vi "HDF5_LogTime.vi"(8 "error in (no error)":errorcluster, 9 "Timestamp":dbl, 10 "TimeStamp_dset":T1 format="%.0x") -> (0 "error out":errorcluster, 2 "date/time string":string, 3 "current time":timestamp)   [LabVIEW 2018]
uses:
  <vilib>/addons/h5labview2/base/hid_t.ctl
  lib_path_mod_20200519.vi
  <vilib>/addons/h5labview2/base/H5Equery.vi
  <vilib>/addons/h5labview2/dataset/H5Dwrite.llb/H5Dwrite.xnode
  <vilib>/addons/h5labview2/dataset/H5D.lvlib
  <vilib>/addons/h5labview2/space/H5S.lvlib
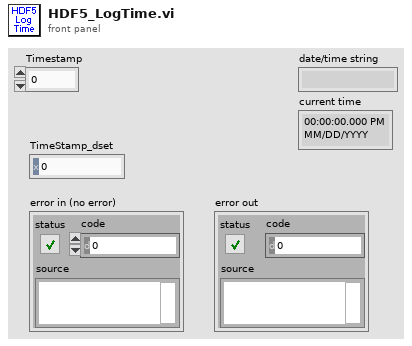
[diagram p1: front panel]
types:
  T1 = typedef "hid_t.ctl" = i32
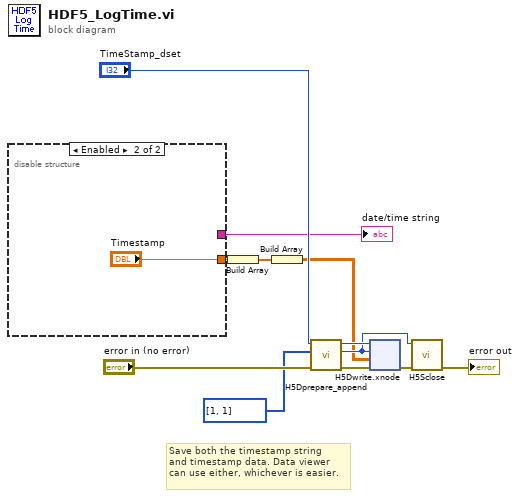
[diagram p0: block diagram]
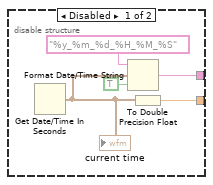
[diagram p2: hidden frame]
diagram:
  # "Save both the timestamp string\nand timestamp data. Data viewer\ncan use either, whichever is easier."
  n1 = disable-structure shown="Enabled" {
    disable-tunnel: [w14 "Timestamp"] -> w4
    disable-tunnel: [w13 _] -> w2
    frame Disabled {
      n2 = Get Date/Time In Seconds() -> (seconds since 1Jan1904=w16:timestamp)
      "current time" <- w16
      n3 = Format Date/Time String(time format string (%c)="%y_%m_%d_%H_%M_%S", seconds (now)=w16, UTC format=TRUE) -> (date/time string=w13:string)
      n4 = To Double Precision Float(number=w16) -> (double precision float=w14:dbl)
    }
    frame Enabled {
    }
  }
  "date/time string" <- w2
  n5 = Build Array(w4) -> (w5:dbl[])
  n6 = Build Array(w5) -> (w3:dbl[][])
  n7 = call <vilib>:"H5Dprepare_append.vi"("error in (no error)"="error in (no error)", "append dims"=i32[] [1, 1] ("size(s)"), "dset in"="TimeStamp_dset") -> ("error out"=w6:errorcluster, "space out"=w8:T1, "dset out"=w9:T1)  [unwired: 5 in, 1 out]
  n8 = xnode "H5Dwrite.xnode"("error in (no error)"=w6, "data"=w3, "file space"=w8, "ref in"=w9) -> ("error out"=w7:errorcluster)  [unwired: 3 in, 2 out]
  n9 = call <vilib>:"H5Sclose.vi"("error in (no error)"=w7, "space in"=w8) -> ("error out"=→"error out":errorcluster)  [unwired: 9 in]
